vi "Create and configure an FPGA Addon.vi"() -> ()   [LabVIEW 2018]
uses:
  <vilib>/addons/VeriStand Custom Device Scripting APIs/FPGA Addon/Scripting API.lvlibp/APIs/Scripting API/TypeDefs/Output Scalar Data.ctl
  <vilib>/addons/VeriStand Custom Device Scripting APIs/FPGA Addon/Scripting API.lvlibp/Addon/Addon Shared/Types/Data Type.ctl
  <vilib>/addons/VeriStand Custom Device Scripting APIs/FPGA Addon/Scripting API.lvlibp
  <vilib>/addons/VeriStand Custom Device Scripting APIs/FPGA Addon/Scripting API.lvlibp/Addon/Addon Shared/FPGA Addon Shared.lvlib
panel:
  out "RIO resource":string
  out "bitfile scalars out":T1[](array[typedef])
  out "FPGA bitfile path":path
  out "error out":errorcluster
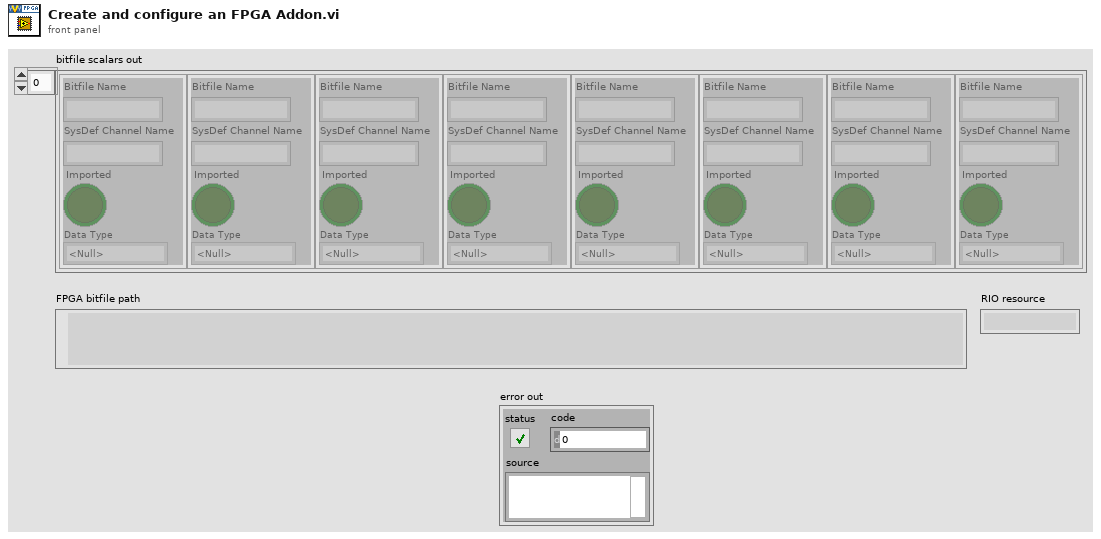
[diagram p1: front panel]
types:
  T1 = typedef "Scripting API.lvlibp/Output Scalar Data.ctl" = cluster{"Bitfile Name":string, "SysDef Channel Name":string, "Imported":bool, "Data Type":T2}
  T2 = typedef "Scripting API.lvlibp/FPGA Addon Shared.lvlib/Data Type.ctl" = enum8{"<Null>", "I8", "I16", "I32", "I64", "U8", "U16", "U32", "U64", "SGL", "Boolean", "Analog PWM In Settings", "Analog PWM In", "Digital PWM In Settings", "Digital PWM In", "Digital PWM Out", "Sine Out", "FXP+/-24.5", "FXP+/-16.5", "FXP+/-32.8", "FXP+/-64.32", "FXP+/-16.7", "FXP+/-20.5", "FXP+/-27.5", "FXP+/-32.16", "FXP+16.3", "FXP+18.3", "Digital Static In", "Digital Static Out", "Digital Static In Settings", "Digital WSS Out", "Quad Encoder Settings", "Quad Encoder In", "Group"}
  T3 = typedef "Scripting API.lvlibp/Custom Device API.lvlib/Custom Device Item Ref.ctl" = u64
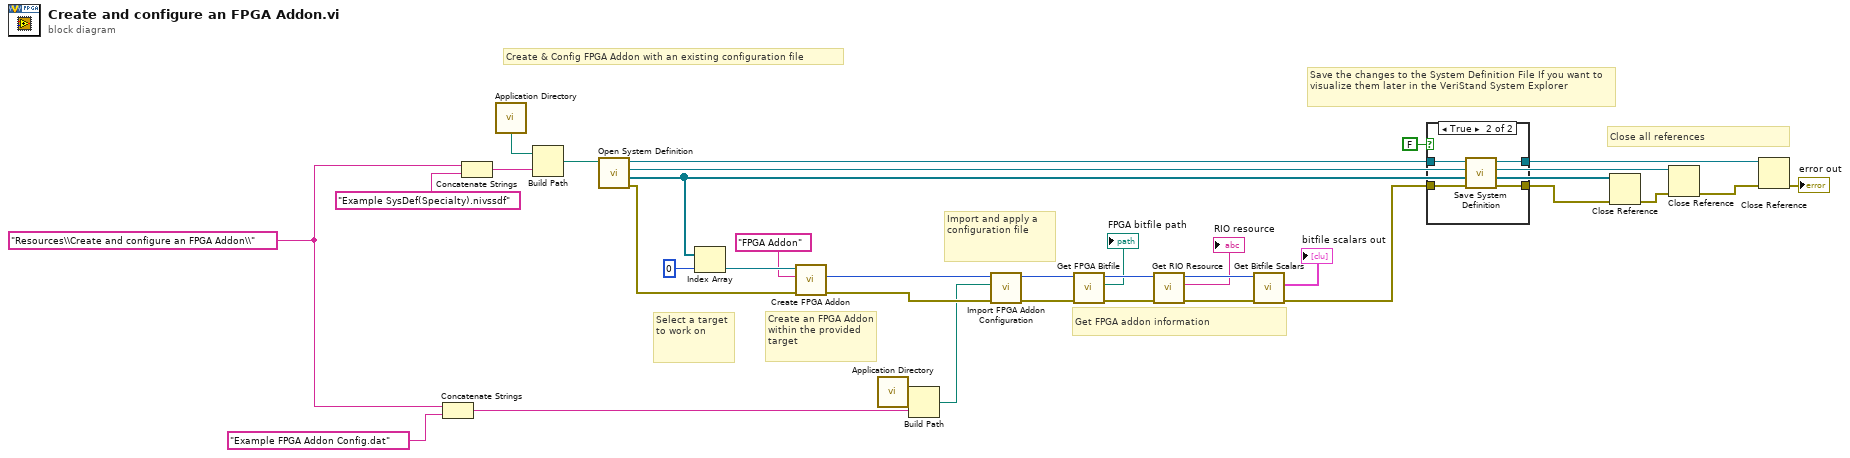
[diagram p0: block diagram]
diagram:
  w14 = "Resources\\Create and configure an FPGA Addon\\" ("name or relative path")
  # "Get FPGA addon information"
  # "Create & Config FPGA Addon with an existing configuration file"
  # "Import and apply a configuration file"
  # "Save the changes to the System Definition File If you want to visualize them later in the VeriStand System Explorer"
  # "Close all references"
  # "Create an FPGA Addon within the provided target"
  # "Select a target to work on"
  n1 = Concatenate Strings(w14, "Example FPGA Addon Config.dat" ("name or relative path")) -> (w12:string)
  n2 = Concatenate Strings(w14, "Example SysDef(Specialty).nivssdf" ("name or relative path")) -> (w15:string)
  n3 = call <vilib>:"Application Directory.vi"() -> ("Application Directory"=w29:path)
  n4 = Build Path(base path=w29, name or relative path=w15) -> (appended path=w28:path)
  n5 = call "Open System Definition.vi"("System Definition File"=w28) -> ("error out"=w20:errorcluster, "targets refnums"=w32:refnum<k24>[], "root refnum"=w33:refnum<k24>, "system definition refnum"=w26:refnum<k24>)  [unwired: 7 in]
  n6 = Index Array(array=w32, index=0) -> (element=w22:refnum<k24>)
  n7 = call <vilib>:"Create FPGA Addon.vi"("error in"=w20, "FPGA addon name"="FPGA Addon" ("fpga addon name"), "target in"=w22) -> ("error out"=w19:errorcluster, "FPGA addon refnum"=w18:T3)  [unwired: 6 in, 1 out]
  n8 = call <vilib>:"Application Directory.vi"() -> ("Application Directory"=w23:path)
  n9 = Build Path(base path=w23, name or relative path=w12) -> (appended path=w17:path)
  n10 = call <vilib>:"Import FPGA Addon Configuration.vi"("error in"=w19, "configuration file path"=w17, "FPGA addon refnum in"=w18) -> ("error out"=w10:errorcluster, "FPGA addon refnum out"=w9:T3)  [unwired: 7 in]
  n11 = call <vilib>:"Get FPGA Bitfile.vi"("error in"=w10, "FPGA addon refnum in"=w9) -> ("error out"=w7:errorcluster, "FPGA bitfile path"=→"FPGA bitfile path":path, "FPGA addon refnum out"=w8:T3)  [unwired: 7 in]
  n12 = call <vilib>:"Get RIO Resource.vi"("error in"=w7, "FPGA addon refnum in"=w8) -> ("error out"=w4:errorcluster, "RIO resource"=→"RIO resource":string, "FPGA addon refnum out"=w5:T3)  [unwired: 7 in]
  n13 = call <vilib>:"Get Bitfile Scalars.vi"("error in"=w4, "FPGA addon refnum in"=w5) -> ("error out"=w3:errorcluster, "bitfile scalars out"=→"bitfile scalars out":T1[])  [unwired: 7 in, 1 out]
  n14 = case shown="True" FALSE {
    tunnel: w26 -> [w36 w40]
    tunnel: [w36 w39] -> w25
    tunnel: [w35 w38] -> w24
    tunnel: w3 -> [w35 w37]
    frame False {
    }
    frame True {
      n15 = call "Save System Definition.vi"("error in (no error)"=w37, ".NET Refnum in"=w40) -> ("error out"=w38:errorcluster, ".NET Refnum out"=w39:refnum<k24>)  [unwired: 8 in]
    }
  }
  n16 = Close Reference(reference=w32, error in (no error)=w24) -> (error out=w31:errorcluster)
  n17 = Close Reference(reference=w33, error in (no error)=w31) -> (error out=w30:errorcluster)
  n18 = Close Reference(reference=w25, error in (no error)=w30) -> (error out=→"error out":errorcluster)
